vi "ADCP_write_parameter_to_serial_port.vi"(0 "ADCP In":refnum<class "ADCP.lvclass">, 1 "Transmit count":u32, 5 "Parameter name":string, 7 "Parameter value":string, 9 "Parameter Index":i32=-1, 11 "error in (no error)":errorcluster, 12 "Transmit interval (ms)":u32) -> (4 "ADCP out":refnum<class "ADCP.lvclass">, 6 "Processed bytes":u8[](array[numeric]), 8 "Data Packet out":T2, 15 "error out":errorcluster)   [LabVIEW 2017, in "ADCP.lvclass"]
uses:
  ADCP.lvclass
  ADCP_Data_Packet_Transmit_Mode.ctl
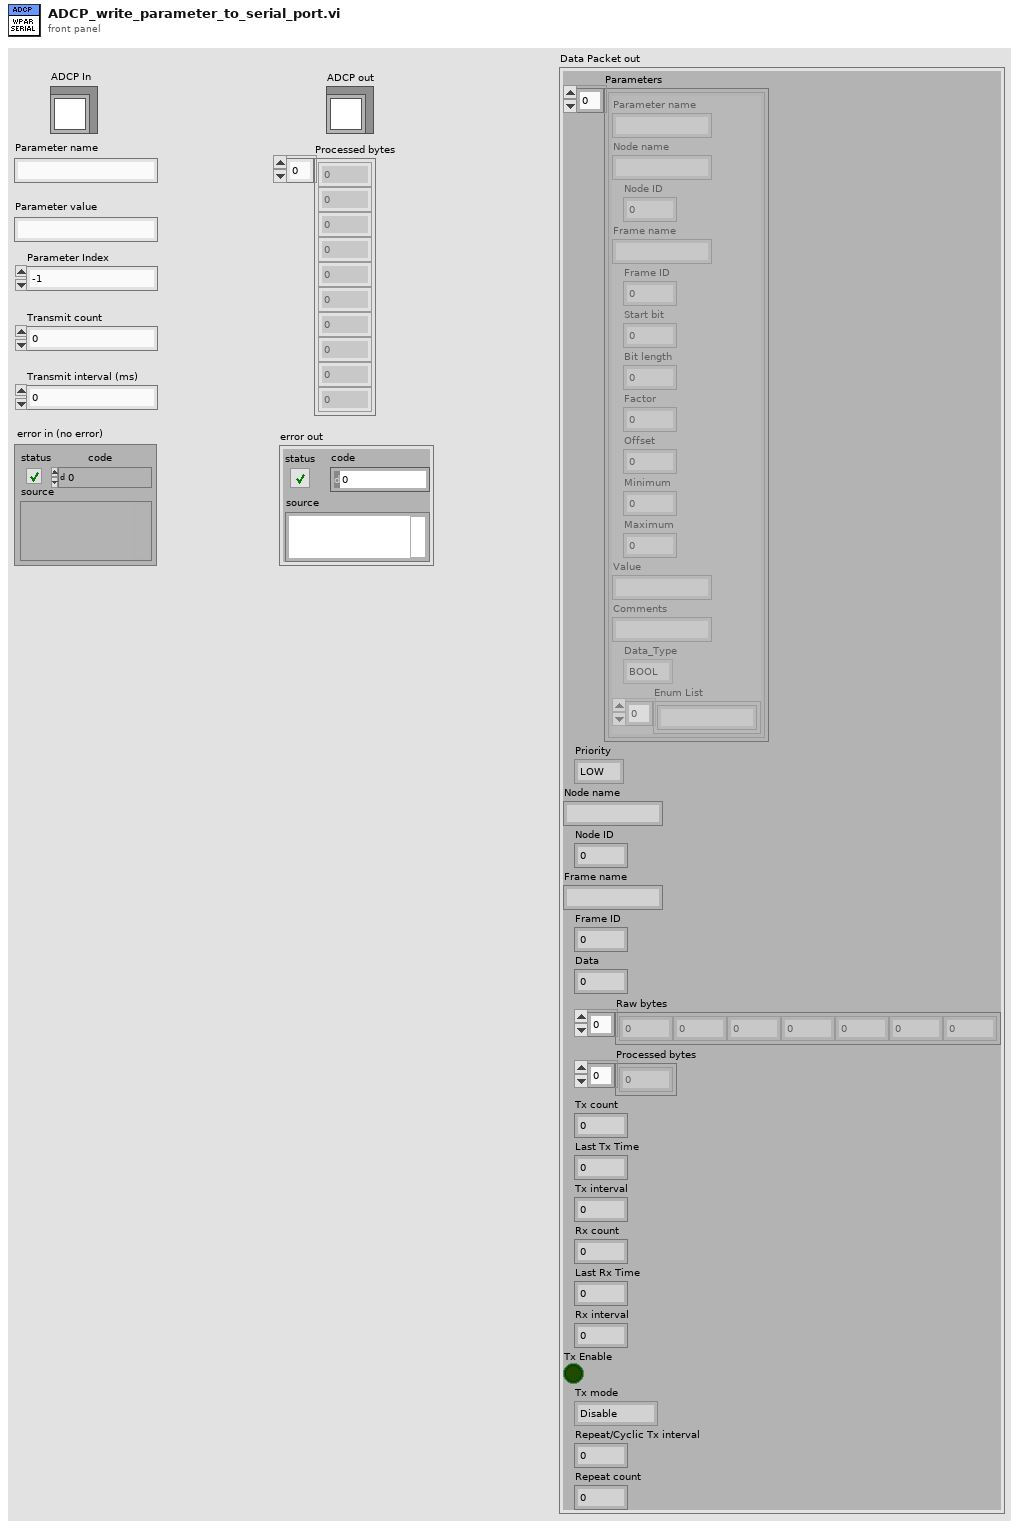
[diagram p1: front panel]
types:
  T1 = typedef "ADCP.lvclass/ADCP_Data_Packet_Transmit_Mode.ctl" = enum16{"Disable", "Single", "Cyclic", "Repeat"}
  T2 = cluster{"Parameters":cluster{"Parameter name":string, "Node name":string, "Node ID":u8, "Frame name":string, "Frame ID":u8, "Start bit":u32, "Bit length":u32, "Factor":dbl, "Offset":dbl, "Minimum":dbl, "Maximum":dbl, "Value":string, "Comments":string, "Data_Type":enum16{"BOOL", "UNSIGNED", "SIGNED", "FLOAT32", "ENUM"}, "Enum List":string[]}[], "Priority":enum16{"LOW", "HIGH"}, "Node name":string, "Node ID":u8, "Frame name":string, "Frame ID":u8, "Data":u32, "Raw bytes":u8[], "Processed bytes":u8[], "Tx count":i32, "Last Tx Time":u32, "Tx interval":u32, "Rx count":i32, "Last Rx Time":u32, "Rx interval":u32, "Tx Enable":bool, "Tx mode":T1, "Repeat/Cyclic Tx interval":u32, "Repeat count":u16}
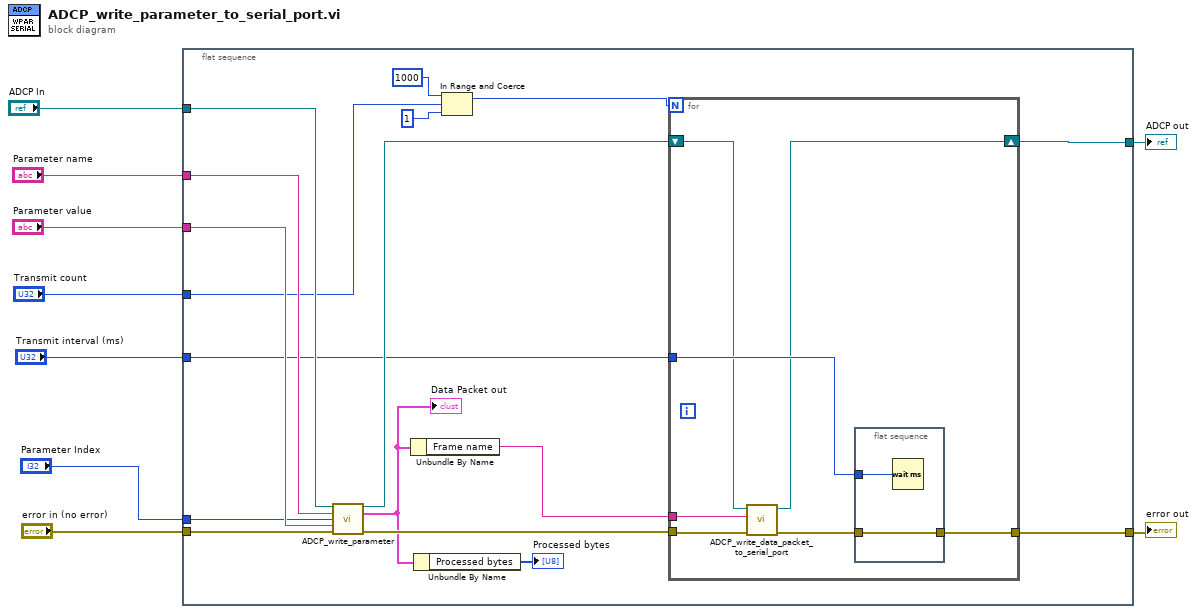
[diagram p0: block diagram]
diagram:
  n1 = flat-sequence {
    tunnel: "ADCP In" -> [w25]
    tunnel: "Parameter name" -> [w24]
    tunnel: "Transmit count" -> [w15]
    tunnel: "Transmit interval (ms)" -> [w20]
    tunnel: "error in (no error)" -> [w26]
    tunnel: "Parameter value" -> [w23]
    tunnel: [w19] -> w3
    tunnel: "Parameter Index" -> [w18]
    tunnel: [w17] -> w1
    frame #0 {
      n2 = call "ADCP_write_parameter.vi"("ADCP in"=w25, "Parameter Name"=w24, "Parameter Index"=w18, "Parameter Value"=w23, "error in (no error)"=w26) -> ("ADCP out"=w21:refnum<class "ADCP.lvclass">, "Data Packet out"=w11:T2, "error out"=w22:errorcluster)  [unwired: 8 in]
      "Data Packet out" <- w11
      n3 = Unbundle By Name(w11) -> ("Frame name"=w16:string)
      n4 = Unbundle By Name(w11) -> ("Processed bytes"=→"Processed bytes":u8[])
      n5 = In Range and Coerce(upper limit=u32 1000, x=w15, lower limit=u32 1) -> (coerced(x)=w14:u32)  [unwired: 1 out]
      n6 = for {
        N: w14 -> [_]
        tunnel: w22 -> [w32]
        shift-right: [w28] -> w19
        shift-left: w21 -> [w29]
        tunnel: w20 -> [w33]
        tunnel: [w30] -> w17
        tunnel: w16 -> [w27]
        n7 = call "ADCP_write_data_packet_to_serial_port.vi"("error in (no error)"=w32, "Frame name"=w27, "ADCP in"=w29) -> ("error out"=w31:errorcluster, "ADCP out"=w28:refnum<class "ADCP.lvclass">)  [unwired: 7 in]
        n8 = flat-sequence {
          tunnel: w33 -> [w35]
          tunnel: w31 -> [w34]
          tunnel: [w34] -> w30
          frame #0 {
            n9 = Wait (ms)(milliseconds to wait=w35) -> ()  [unwired: 1 out]
          }
        }
      }
    }
  }
  "error out" <- w1
  "ADCP out" <- w3
